vi "数值转换为U16.vi"(10 "数值数组输入":enum16{"0", "1"}[][](array[ring])) -> (2 "U16输出":u16[](array[numeric]))   [LabVIEW 2010]
panel:
  # "将数据索引号和数据值转换为U16"
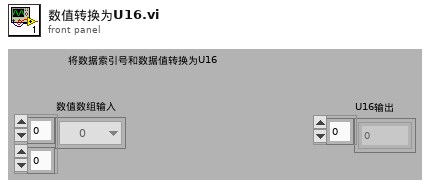
[diagram p1: front panel]
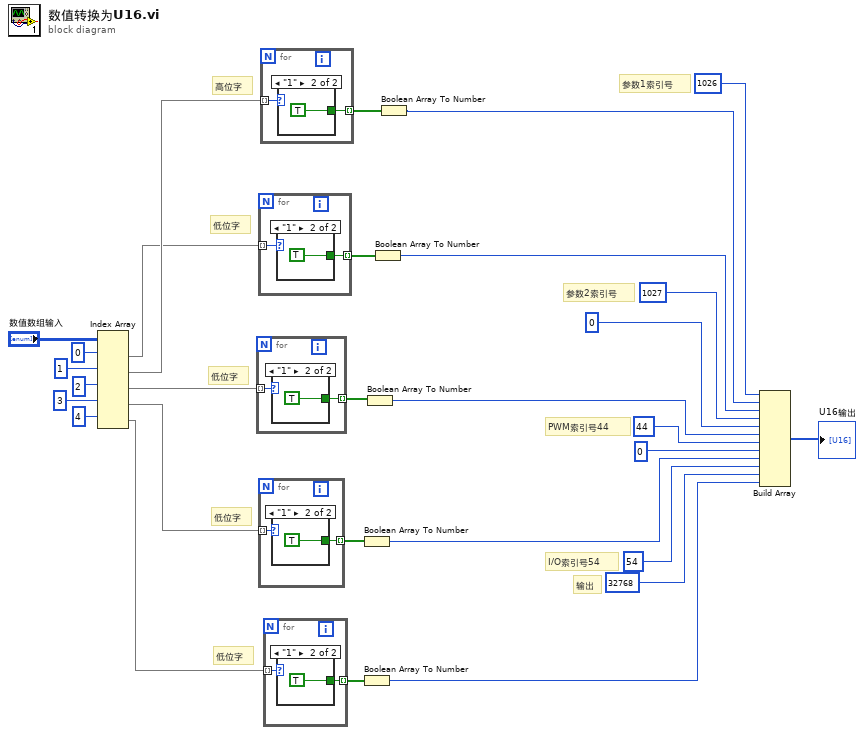
[diagram p0: block diagram]
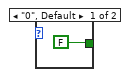
[diagram p2: hidden frame]
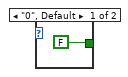
[diagram p3: hidden frame]
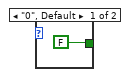
[diagram p4: hidden frame]
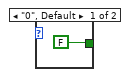
[diagram p5: hidden frame]
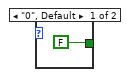
[diagram p6: hidden frame]
diagram:
  # "低位字"
  # "低位字"
  # "低位字"
  # "低位字"
  # "高位字"
  # "输出"
  # "I/O索引号54"
  # "PWM索引号44"
  # "参数2索引号"
  # "参数1索引号"
  n1 = Index Array(array="数值数组输入", index (row) #1=0 ("索引 (行)"), index (row) #2=1 ("索引 (行)"), index (row) #3=2 ("索引 (行)"), index (row) #4=3 ("索引 (行)"), index (row) #5=4 ("索引 (行)")) -> (element #1=w1:enum16{"0", "1"}[], element #2=w2:enum16{"0", "1"}[], element #3=w23:enum16{"0", "1"}[], element #4=w22:enum16{"0", "1"}[], element #5=w21:enum16{"0", "1"}[])  [unwired: 5 in]
  n2 = for {
    tunnel: w23 -> [w31] mode=indexing
    tunnel: [w30] -> w6 mode=indexing
    n3 = case shown="\"1\"" w31 {
      tunnel: [FALSE TRUE] -> w30
      frame "0", Default {
      }
      frame "1" {
      }
    }
  }
  n4 = for {
    tunnel: w1 -> [w35] mode=indexing
    tunnel: [w34] -> w11 mode=indexing
    n5 = case shown="\"1\"" w35 {
      tunnel: [FALSE TRUE] -> w34
      frame "0", Default {
      }
      frame "1" {
      }
    }
  }
  n6 = for {
    tunnel: w22 -> [w39] mode=indexing
    tunnel: [w38] -> w8 mode=indexing
    n7 = case shown="\"1\"" w39 {
      tunnel: [FALSE TRUE] -> w38
      frame "0", Default {
      }
      frame "1" {
      }
    }
  }
  n8 = for {
    tunnel: w2 -> [w43] mode=indexing
    tunnel: [w42] -> w12 mode=indexing
    n9 = case shown="\"1\"" w43 {
      tunnel: [FALSE TRUE] -> w42
      frame "0", Default {
      }
      frame "1" {
      }
    }
  }
  n10 = for {
    tunnel: w21 -> [w47] mode=indexing
    tunnel: [w46] -> w10 mode=indexing
    n11 = case shown="\"1\"" w47 {
      tunnel: [FALSE TRUE] -> w46
      frame "0", Default {
      }
      frame "1" {
      }
    }
  }
  n12 = Boolean Array To Number ("布尔数组至数值转换")(Boolean array=w8) -> (number=w7:u16)
  n13 = Boolean Array To Number ("布尔数组至数值转换")(Boolean array=w10) -> (number=w9:u16)
  n14 = Boolean Array To Number ("布尔数组至数值转换")(Boolean array=w6) -> (number=w5:u16)
  n15 = Boolean Array To Number ("布尔数组至数值转换")(Boolean array=w11) -> (number=w4:u16)
  n16 = Boolean Array To Number ("布尔数组至数值转换")(Boolean array=w12) -> (number=w3:u16)
  n17 = Build Array(u16 1026, w3, w4, u16 1027, u16 0 ("数值_U16_0"), w5, u16 44, u16 0 ("数值_U16_0"), w7, u16 54, u16 32768 ("数值_U16_0"), w9) -> (→"U16输出":u16[])
